vi "ReplaceMarkers.vi"(8 "Owner":u8=255, 9 "Color":u32(colorbox)=32639, 10 "Pixels 3":dbl[][](array[numeric]), 11 "MarkersArray":T1) -> (0 "Owner Out":u8=255, 3 "MarkersArray Out":T1)   [LabVIEW 2017, in "ImageAcquisitionLibrary.lvlib"]
uses:
  ImageAcquisitionLibrary.lvlib
  MarkersArray.ctl
  Marker.ctl
panel:
  out "size(s)":i32
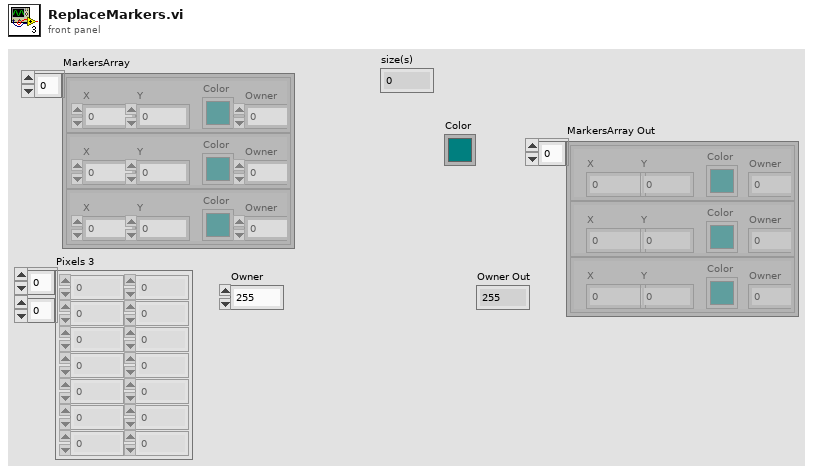
[diagram p1: front panel]
types:
  T1 = typedef "ImageAcquisitionLibrary.lvlib/MarkersArray.ctl" = T2[]
  T2 = typedef "ImageAcquisitionLibrary.lvlib/Marker.ctl" = cluster{"X":dbl, "Color":u32, "Y ":dbl, "Owner":u8}
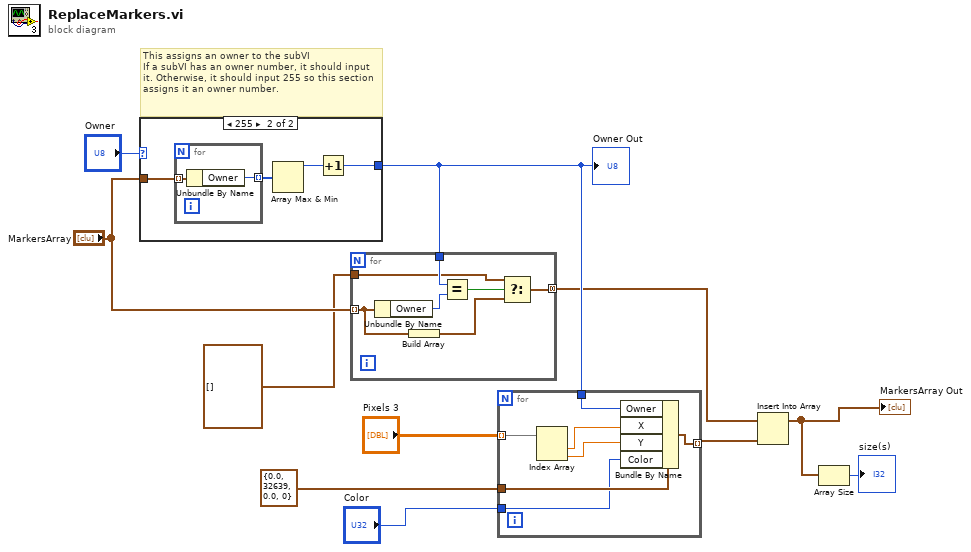
[diagram p0: block diagram]
diagram:
  # "This assigns an owner to the subVI\nIf a subVI has an owner number, it should input it. Otherwise, it should input 255 so this section assigns it an owner number."
  n1 = case shown="255" "Owner" {
    selector: "Owner" -> [w12 _]
    tunnel: "MarkersArray" -> [_ w16]
    tunnel: [w12 w13] -> w6
    frame 0, Default {
    }
    frame 255 {
      n2 = for {
        tunnel: w16 -> [w18] mode=indexing
        tunnel: [w17] -> w15 mode=indexing
        n3 = Unbundle By Name(w18) -> ("Owner"=w17:u8)
      }
      n4 = Array Max & Min(array=w15) -> (max value=w14:u8)  [unwired: 3 out]
      n5 = Increment(x=w14) -> (x+1=w13:u8)
    }
  }
  "Owner Out" <- w6
  n6 = for {
    tunnel: "MarkersArray" -> [w22] mode=indexing
    tunnel: w6 -> [w24]
    tunnel: T1 [] ("MarkersArray") -> [w20]
    tunnel: [w19] -> w4 mode=concatenating
    n7 = Unbundle By Name(w22) -> ("Owner"=w25:u8)
    n8 = Build Array(w22) -> (w21:T2[])
    n9 = Equal?(x=w24, y=w25) -> (x = y?=w23:bool)
    n10 = Select(t=w20, s=w23, f=w21) -> (s? t:f=w19:T1)
  }
  n11 = for {
    tunnel: "Pixels 3" -> [w31] mode=indexing
    tunnel: T2 {"X"=0.0, "Color"=32639, "Y "=0.0, "Owner"=0} ("Marker") -> [w32]
    tunnel: "Color" -> [w28]
    tunnel: [w27] -> w9 mode=indexing
    tunnel: w6 -> [w26]
    n12 = Index Array(array=w31) -> (element #1=w30:dbl, element #2=w29:dbl)  [unwired: 2 in]
    n13 = Bundle By Name(cluster=w32, "Owner"=w26, "X"=w30, "Y"=w29, "Color"=w28) -> (w27:T2)
  }
  n14 = Insert Into Array(array=w4, new element=w9) -> (w2:T1)  [unwired: 1 in]
  "MarkersArray Out" <- w2
  n15 = Array Size(array=w2) -> (size(s)=→"size(s)":i32)
